vi "TCP test prog.vi"() -> ()   [LabVIEW 2023]
doc: "Demonstrates how to open a connection to an TCP server, read the data being sent, and display the data on a chart. This VI is designed to stop if the TCP connection is terminated."
panel:
  out "?":bool
  out "?":string
  out "?":string
  out "?":string
  out "?":string
  out "?":string
  out "?":string
  in  "Number of channels":dbl
  out "?":string
  out "String 2":string
  in  "Server Closed":string="The server VI closed the connection."
  # "Overview: Demonstrates the use of the TCP functions to connect to a TCP server VI and receive data.\nInstructions:\n1. Ensure Simple TCP - Server.vi is already running.\n2. Run the VI.\n3. Click Stop to stop the VI. Note that if you stop the server VI, this VI will stop automatically."
  # "A0\n\nA1\n\nA2\n\nA3\n\nA4\n\nA5\n\nA6"
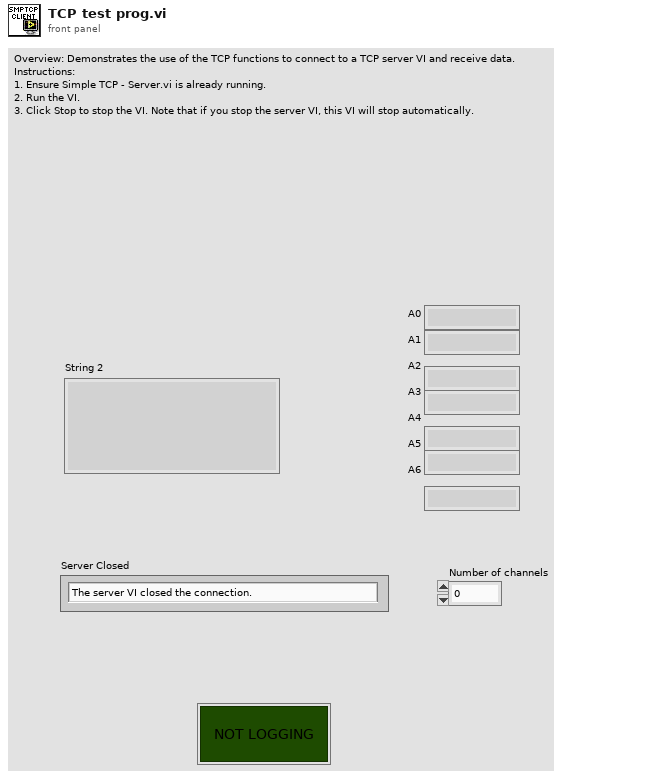
[diagram p1: front panel]
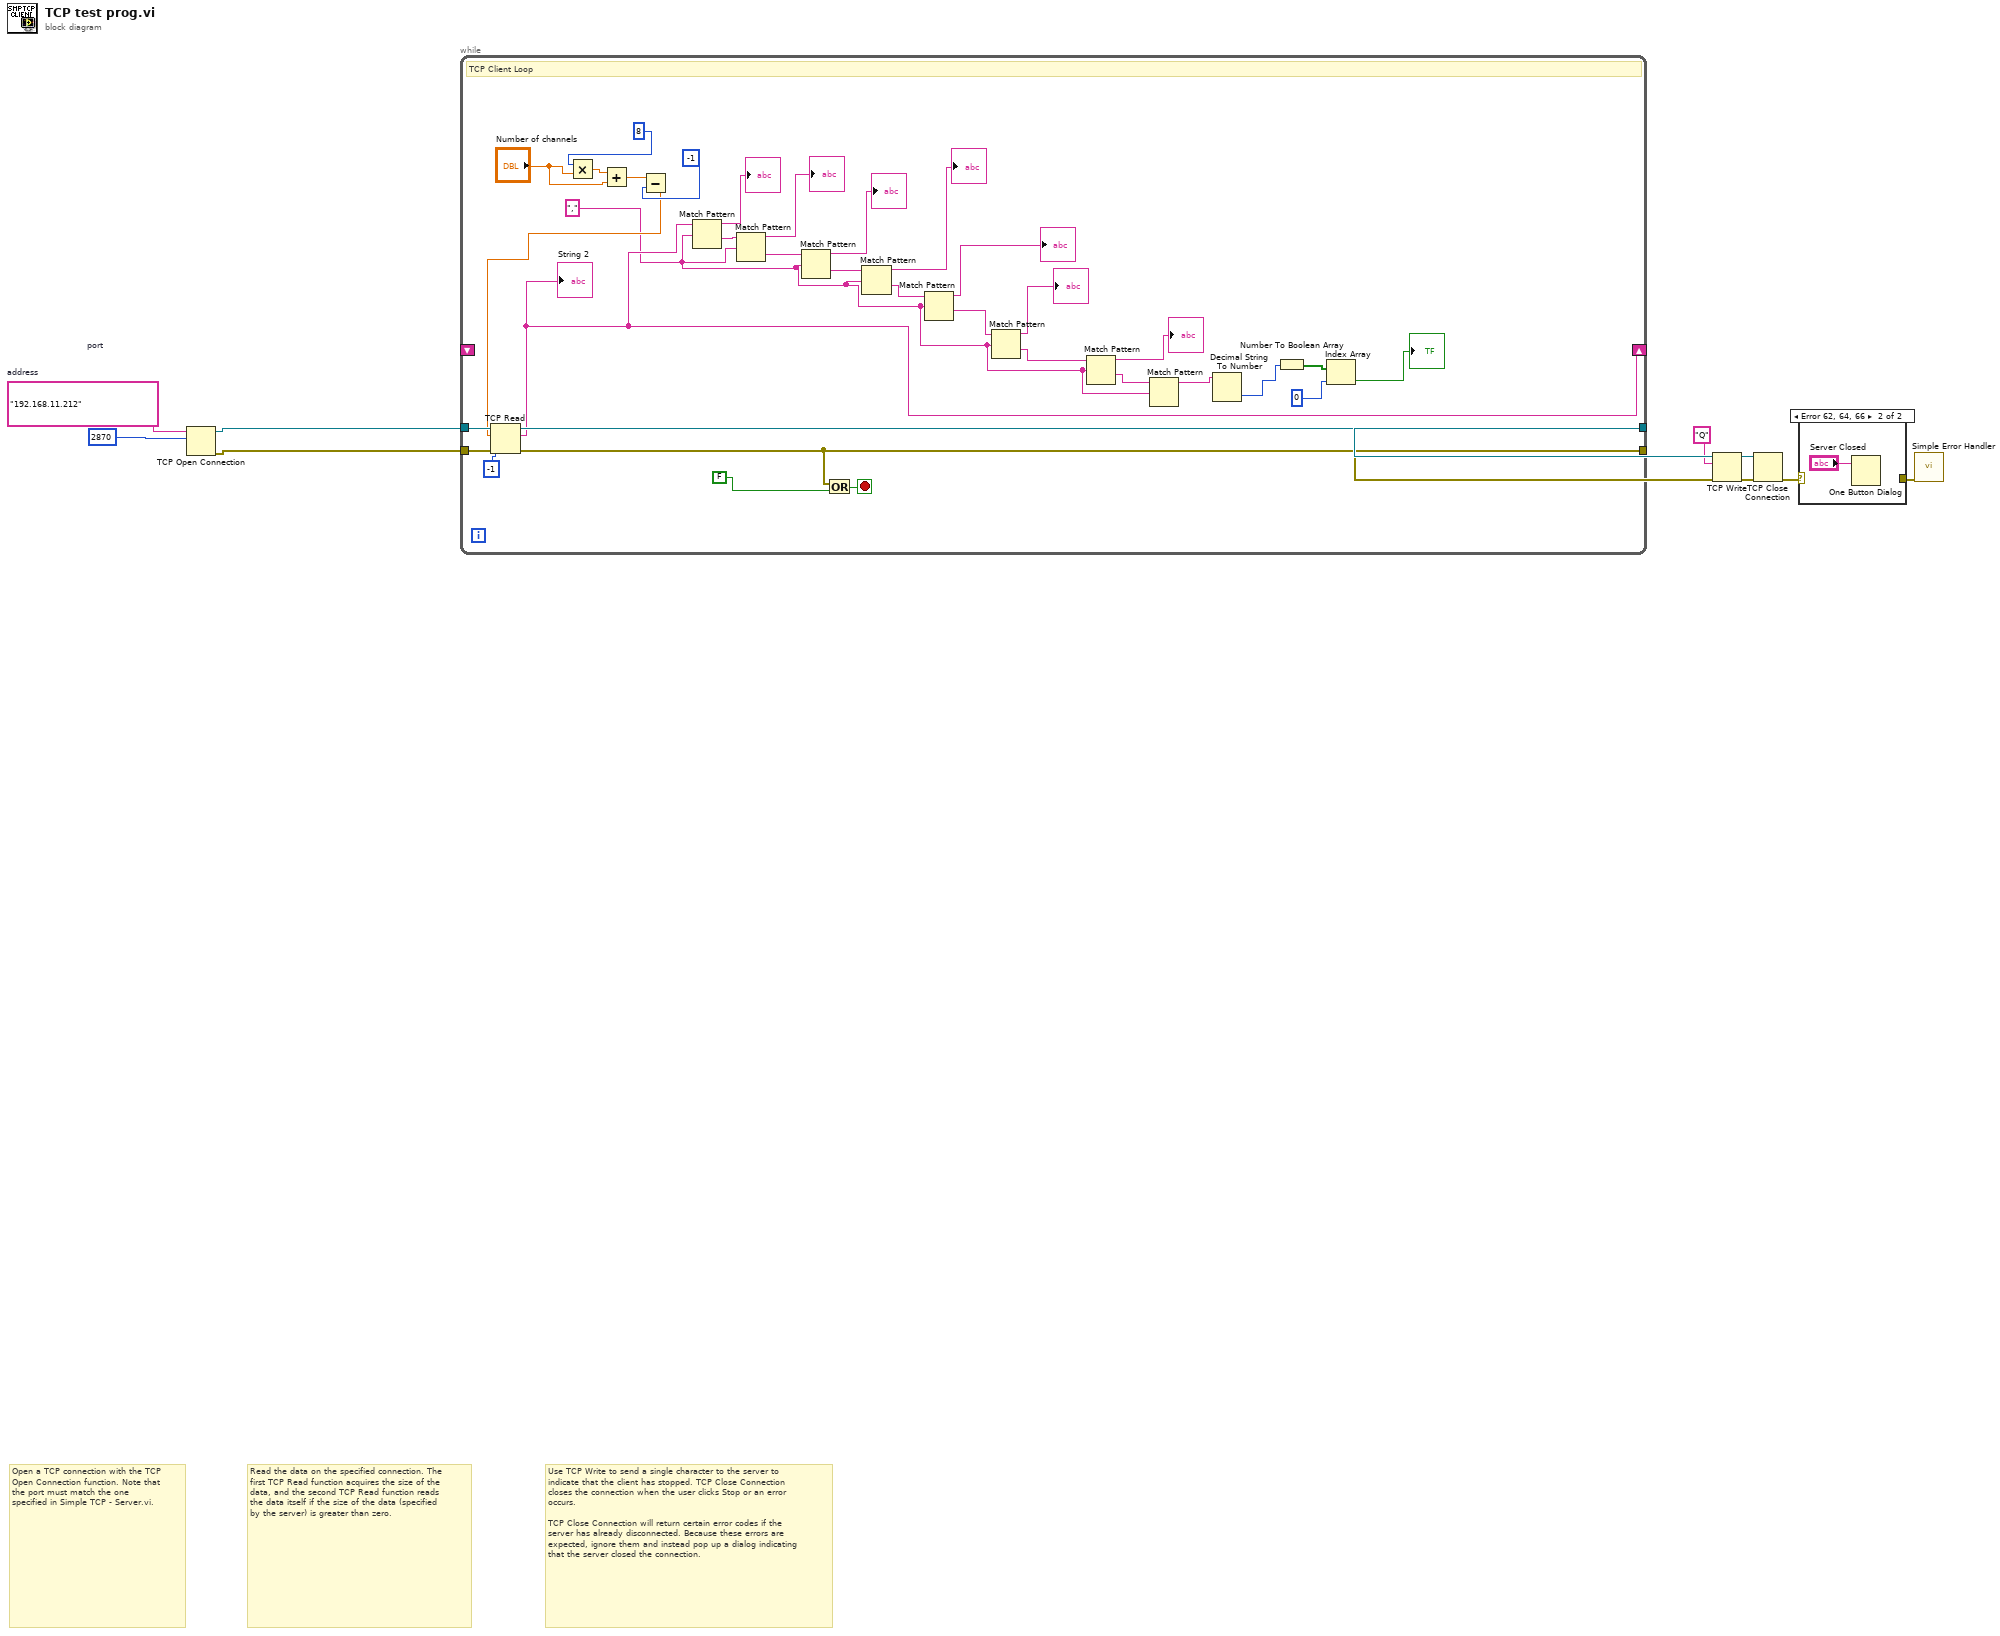
[diagram p0: block diagram]
diagram:
  w1 = u16 2870  # port
  w2 = "192.168.11.212"  # address
  # "Use TCP Write to send a single character to the server to indicate that the client has stopped. TCP Close Connection closes the connection when the user clicks Stop or an error occurs.\n\nTCP Close Connection will return certain error codes if the server has already disconnected. Because these errors are expected, ignore them and instead pop up a dialog indicating that the server closed the connection."
  # "Read the data on the specified connection. The first TCP Read function acquires the size of the data, and the second TCP Read function reads the data itself if the size of the data (specified by the server) is greater than zero."
  # "Open a TCP connection with the TCP Open Connection function. Note that the port must match the one specified in Simple TCP - Server.vi."
  n1 = TCP Open Connection(address=w2, remote port or service name=w1) -> (connection ID=w11:refnum<k5>, error out=w10:errorcluster)  [unwired: 3 in]
  n2 = while {
    tunnel: w10 -> [w44]
    tunnel: w11 -> [w45]
    tunnel: [w41] -> w8
    tunnel: [w40] -> w6
    shift-right: [w39] -> _
    shift-left: _ -> [_]
    stop <- w43 stop-if-true
    w17 = ","
    # "TCP Client Loop"
    n3 = Multiply(x=8, y="Number of channels") -> (x*y=w29:dbl)
    n4 = Add(x=w29, y="Number of channels") -> (x+y=w28:dbl)
    n5 = Subtract(x=w28, y=-1) -> (x-y=w26:dbl)
    n6 = TCP Read(connection ID=w45, bytes to read=w26, error in (no error)=w44, 9:-1 ("timeout ms (25000)")) -> (connection ID out=w41:refnum<k5>, data out=w39:string, error out=w40:errorcluster)  [unwired: 1 in]
    "String 2" <- w39
    n7 = Match Pattern(string=w39, regular expression=w17) -> (before substring=→"?":string, after substring=w36:string)  [unwired: 1 in, 2 out]
    n8 = Match Pattern(string=w36, regular expression=w17) -> (before substring=→"?":string, after substring=w34:string)  [unwired: 1 in, 2 out]
    n9 = Match Pattern(string=w34, regular expression=w17) -> (before substring=→"?":string, after substring=w32:string)  [unwired: 1 in, 2 out]
    n10 = Or(x=w40, y=FALSE) -> (x .or. y?=w43:bool)
    n11 = Match Pattern(string=w32, regular expression=w17) -> (before substring=→"?":string, after substring=w24:string)  [unwired: 1 in, 2 out]
    n12 = Match Pattern(string=w24, regular expression=w17) -> (before substring=→"?":string, after substring=w22:string)  [unwired: 1 in, 2 out]
    n13 = Match Pattern(string=w22, regular expression=w17) -> (before substring=→"?":string, after substring=w20:string)  [unwired: 1 in, 2 out]
    n14 = Match Pattern(string=w20, regular expression=w17) -> (before substring=→"?":string, after substring=w18:string)  [unwired: 1 in, 2 out]
    n15 = Match Pattern(string=w18, regular expression=w17) -> (before substring=w15:string)  [unwired: 1 in, 3 out]
    n16 = Decimal String To Number(string=w15) -> (number=w13:i32)  [unwired: 2 in, 1 out]
    n17 = Number To Boolean Array(number=w13) -> (Boolean array=w16:bool[])
    n18 = Index Array(array=w16, index=0) -> (element=→"?":bool)
  }
  n19 = TCP Write(connection ID=w8, data in="Q", error in (no error)=w6) -> (connection ID out=w9:refnum<k5>, error out=w7:errorcluster)  [unwired: 2 out]
  n20 = TCP Close Connection(connection ID=w9, error in (no error)=w7) -> (error out=w4:errorcluster)  [unwired: 1 in, 1 out]
  n21 = case shown="Error 62, 64, 66" w4 {
    selector: w4 -> [w46 _]
    tunnel: [w46 _] -> w3
    frame #0 {
    }
    frame #1 {
      n22 = One Button Dialog(message="Server Closed") -> ()  [unwired: 1 in, 1 out]
    }
  }
  n23 = call <vilib>:"Simple Error Handler.vi"("error in (no error)"=w3) -> ()  [unwired: 4 in, 5 out]
